vi "GetGraphSettings.vi"(8 "Error In":errorcluster, 11 "Setting's name":string) -> (0 "Error Out":errorcluster, 3 "Result":string)   [LabVIEW 2018]
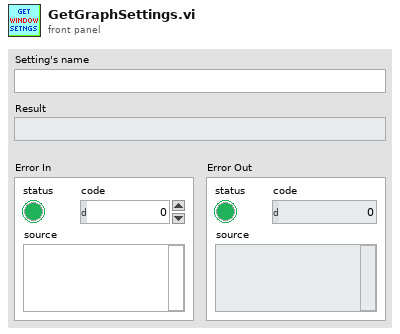
[diagram p1: front panel]
types:
  T1 = enum16{"open", "replace", "create", "open or create", "replace or create", "replace or create with confirmation"}
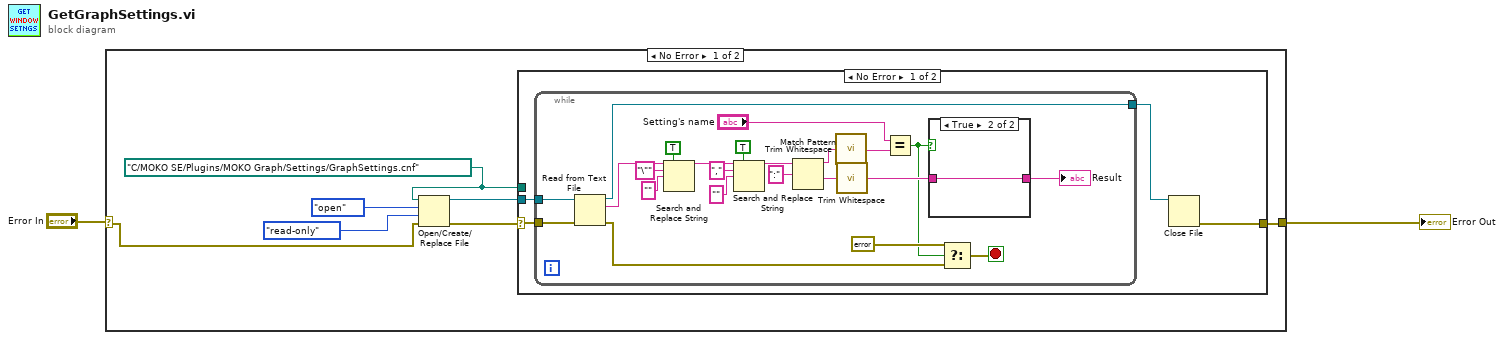
[diagram p0: block diagram]
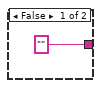
[diagram p2: hidden frame]
diagram:
  n1 = case shown="No Error" "Error In" {
    selector: "Error In" -> [w3 w40]
    tunnel: [w4 w40] -> w1
    frame No Error {
      w6 = path "C:/MOKO SE/Plugins/MOKO Graph/Settings/GraphSettings.cnf" ("file path (use dialog)")
      n2 = Open/Create/Replace File(file path (use dialog)=w6, error in=w3, operation (0:open)=T1."open", access (0:read/write)=enum16{"read/write", "read-only", "write-only"}."read-only") -> (refnum out=w5:refnum<file>, error out=w7:errorcluster)  [unwired: 2 in, 1 out]
      n3 = case shown="No Error" w7 {
        selector: w7 -> [w11 w39]
        tunnel: w6 -> [_ _]
        tunnel: w5 -> [w13 _]
        tunnel: [w10 w39] -> w4
        frame No Error {
          n4 = while {
            tunnel: w13 -> [w23]
            tunnel: [w22] -> w12
            tunnel: w11 -> [w21]
            stop <- w15 stop-if-true
            n5 = Read from Text File(file (use dialog)=w23, error in=w21) -> (refnum out=w22:refnum<file>, text=w34:string, error out=w16:errorcluster)  [unwired: 2 in, 1 out]
            n6 = Search and Replace String(replace all?=TRUE ("replace all? (F)"), input string=w34, search string="\"", replace string="" ("replace string (\"\")")) -> (result string=w30:string)  [unwired: 4 in, 3 out]
            n7 = Search and Replace String(replace all?=TRUE ("replace all? (F)"), input string=w30, search string=",", replace string="" ("replace string (\"\")")) -> (result string=w26:string)  [unwired: 4 in, 3 out]
            n8 = Match Pattern(string=w26, regular expression=":") -> (before substring=w36:string, after substring=w35:string)  [unwired: 1 in, 2 out]
            n9 = call <vilib>:"Trim Whitespace.vi"("string"=w36) -> ("trimmed string"=w19:string)  [unwired: 1 in]
            n10 = call <vilib>:"Trim Whitespace.vi"("string"=w35) -> ("trimmed string"=w24:string)  [unwired: 1 in]
            n11 = Equal?(x="Setting's name", y=w19) -> (x = y?=w14:bool)
            n12 = case shown="True" w14 {
              tunnel: w24 -> [_ w38]
              tunnel: ["" w38] -> w20
              frame False {
              }
              frame True {
              }
            }
            "Result" <- w20
            n13 = Select(t=errorcluster {"status"=TRUE, "code"=0, "source"=""} ("error out"), s=w14, f=w16) -> (s? t:f=w15:errorcluster)
          }
          n14 = Close File(refnum=w12) -> (error out=w10:errorcluster)  [unwired: 1 in, 1 out]
        }
        frame Error {
        }
      }
    }
    frame Error {
    }
  }
  "Error Out" <- w1
